vi "get valid conv subarray (subVI).vi"(1 "k size":i32, 3 "X * k":dbl[](array[numeric])) -> (0 "X * k valid":dbl[](array[numeric]))   [LabVIEW 2021]
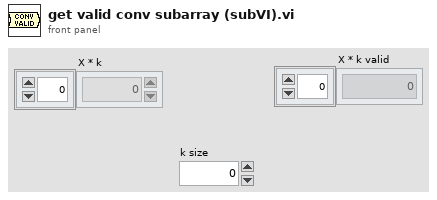
[diagram p1: front panel]
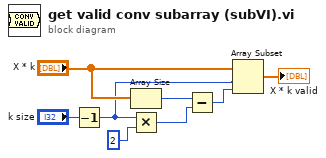
[diagram p0: block diagram]
diagram:
  n1 = Decrement(x="k size") -> (x-1=w3:i32)
  n2 = Array Size(array="X * k") -> (size(s)=w5:i32)
  n3 = Multiply(x=w3, y=2) -> (x*y=w6:i32)
  n4 = Subtract(x=w5, y=w6) -> (x-y=w2:i32)
  n5 = Array Subset(array="X * k", index=w3, length=w2) -> (→"X * k valid":dbl[])
